vi "stop.vi"(11 "Experience ID":string="Test") -> (0 "error out":errorcluster={"status"=TRUE, "code"=2, "source"="incorrect path for Experience ID"})   [LabVIEW 2020]
uses:
  Configuration/Global_Configurations.vi
panel:
  # "Stop"
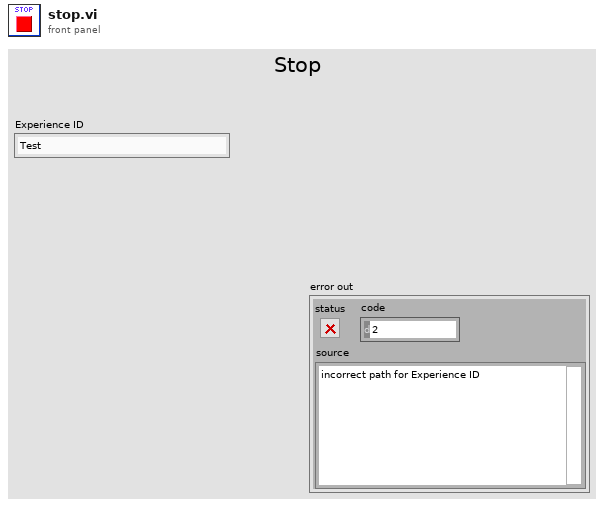
[diagram p1: front panel]
types:
  T1 = enum32{"Bad", "Idle", "Run top level", "Running"}
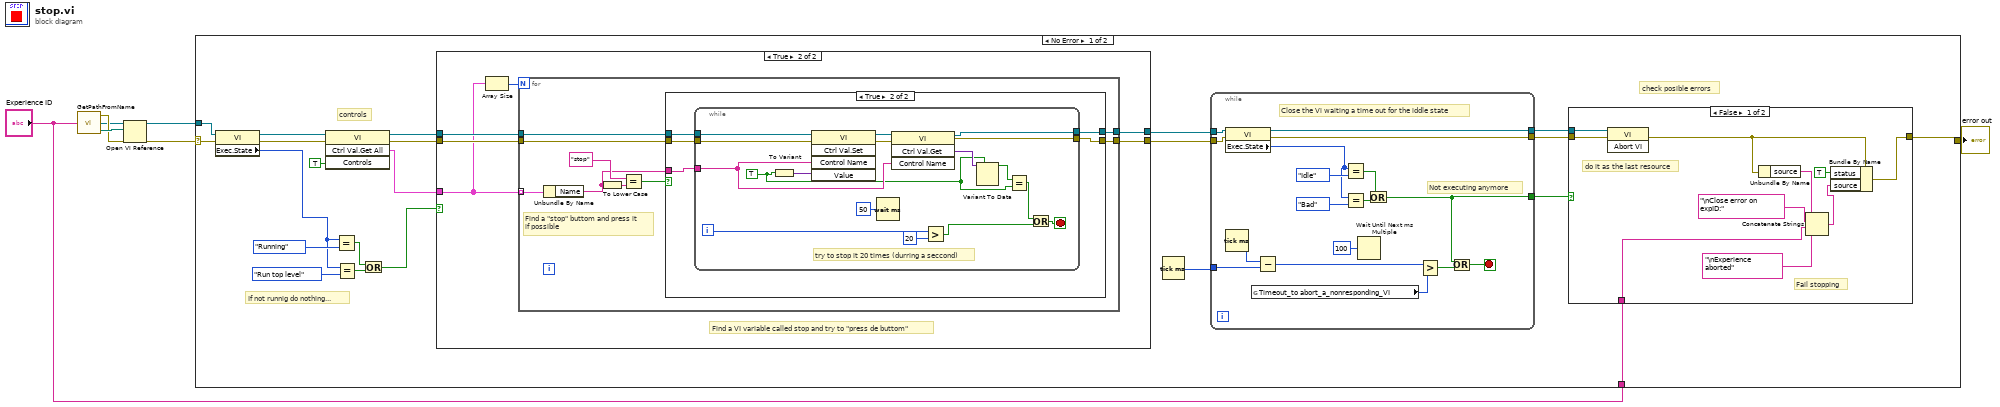
[diagram p0: block diagram]
diagram:
  n1 = call "GetPathFromName.vi"("Experience ID"="Experience ID") -> ("VI_Path"=w7:path, "application reference"=w1:refnum<vi>, "Error out"=w6:errorcluster)  [unwired: 2 in]
  n2 = Open VI Reference(application reference (local)=w1, vi path=w7, error in (no error)=w6) -> (vi reference=w3:refnum<vi>, error out=w4:errorcluster)  [unwired: 3 out]
  n3 = case shown="No Error" w4 {
    selector: w4 -> [w18 w99]
    tunnel: [w15 w99] -> w5
    tunnel: w3 -> [w17 _]
    tunnel: "Experience ID" -> [w14 _]
    frame No Error {
      # "check posible errors"
      # "If not runnig do nothing..."
      # "controls"
      n4 = property class="VI"(reference=w17, error in=w18) -> (reference out=w23:refnum<vi>, error out=w22:errorcluster, "Exec.State"=w16:T1)
      n5 = invoke class="VI" method="Ctrl Val.Get All"(reference=w23, error in=w22, "Controls"=TRUE) -> (reference out=w24:refnum<vi>, error out=w21:errorcluster, "Get All Control Values Variant"=w20:cluster{"Name":string, "Variant Data":variant}[])  [unwired: 1 in, 1 out]
      n6 = Equal?(x=w16, y=T1."Running") -> (x = y?=w28:bool)
      n7 = Equal?(x=w16, y=T1."Run top level") -> (x = y?=w26:bool)
      n8 = Or(x=w28, y=w26) -> (x .or. y?=w19:bool)
      n9 = case shown="True" w19 {
        tunnel: w20 -> [_ w61]
        tunnel: w24 -> [w58 w65]
        tunnel: w21 -> [w59 w64]
        tunnel: [w59 w63] -> w13
        tunnel: [w58 w60] -> w12
        frame False {
        }
        frame True {
          # "Find a VI variable called stop and try to \"press de buttom\""
          n10 = Array Size(array=w61) -> (size(s)=w62:i32)
          n11 = for {
            N: w62 -> [_]
            tunnel: w61 -> [w74] mode=indexing
            tunnel: w65 -> [w72]
            tunnel: w64 -> [w71]
            tunnel: [w69] -> w63
            tunnel: [w66] -> w60
            # "Find a \"stop\" buttom and press it\nif possible"
            n12 = Unbundle By Name(w74) -> ("Name"=w67:string)
            n13 = To Lower Case(string=w67) -> (all lower case string=w68:string)
            n14 = Equal?(x="stop" ("y"), y=w68) -> (x = y?=w73:bool)
            n15 = case shown="True" w73 {
              tunnel: w72 -> [w75 w81]
              tunnel: w71 -> [w76 w80]
              tunnel: [w76 w79] -> w69
              tunnel: w67 -> [_ w78]
              tunnel: [w75 w77] -> w66
              frame False {
              }
              frame True {
                n16 = while {
                  tunnel: w81 -> [w96]
                  tunnel: w80 -> [w98]
                  tunnel: [w83] -> w79
                  tunnel: w78 -> [w88]
                  tunnel: [w82] -> w77
                  i -> [w94]
                  stop <- w95 stop-if-true
                  w85 = TRUE
                  # "try to stop it 20 times (durring a seccond)"
                  n17 = To Variant(anything=w85) -> (Variant=w97:variant)
                  n18 = invoke class="VI" method="Ctrl Val.Set"(reference=w96, error in=w98, "Control Name"=w88, "Value"=w97) -> (reference out=w90:refnum<vi>, error out=w89:errorcluster)  [unwired: 1 in, 3 out]
                  n19 = Wait (ms)(milliseconds to wait=u32 50) -> ()  [unwired: 1 out]
                  n20 = invoke class="VI" method="Ctrl Val.Get"(reference=w90, error in=w89, "Control Name"=w88) -> (reference out=w82:refnum<vi>, error out=w83:errorcluster, "Get Control Value Variant"=w87:variant)  [unwired: 1 in, 1 out]
                  n21 = Greater?(x=w94, y=20) -> (0:w92:bool)
                  n22 = Variant To Data(type=w85, Variant=w87) -> (data=w84:bool)  [unwired: 1 in, 1 out]
                  n23 = Equal?(x=w84, y=w85) -> (x = y?=w86:bool)
                  n24 = Or(x=w86, y=w92) -> (x .or. y?=w95:bool)
                }
              }
            }
          }
        }
      }
      n25 = Tick Count (ms)() -> (millisecond timer value=w11:u32)
      n26 = while {
        tunnel: w12 -> [w46]
        tunnel: [w36] -> w8
        tunnel: [w37] -> w10
        tunnel: [w31] -> w9
        tunnel: w11 -> [w39]
        tunnel: w13 -> [w30]
        stop <- w43 stop-if-true
        # "Not executing anymore"
        # "Close the Vi waiting a time out for the iddle state"
        n27 = property class="VI"(reference=w46, error in=w30) -> (reference out=w36:refnum<vi>, error out=w37:errorcluster, "Exec.State"=w33:T1)
        n28 = Tick Count (ms)() -> (millisecond timer value=w38:u32)
        n29 = global read "Global_Configurations.vi" "Timeout_to abort_a_nonresponding_VI"() -> (w40:u32)
        n30 = Subtract(x=w38, y=w39) -> (x-y=w41:u32)
        n31 = Equal?(x=w33, y=T1."Idle") -> (x = y?=w35:bool)
        n32 = Equal?(x=w33, y=T1."Bad") -> (x = y?=w32:bool)
        n33 = Wait Until Next ms Multiple(millisecond multiple=u32 100) -> ()  [unwired: 1 out]
        n34 = Or(x=w35, y=w32) -> (x .or. y?=w31:bool)
        n35 = Greater?(x=w41, y=w40) -> (0:w42:bool)
        n36 = Or(x=w31, y=w42) -> (x .or. y?=w43:bool)
      }
      n37 = case shown="False" w9 {
        tunnel: [w56 w57] -> w15
        tunnel: w10 -> [w48 w57]
        tunnel: w14 -> [w51 _]
        tunnel: w8 -> [w49 _]
        frame False {
          # "do it as the last resource"
          # "Fail stopping"
          n38 = invoke class="VI" method="Abort VI"(reference=w49, error in=w48) -> (error out=w50:errorcluster)  [unwired: 1 in, 2 out]
          n39 = Unbundle By Name(w50) -> ("source"=w53:string)
          n40 = Concatenate Strings(w53, "\nClose error on expID:" ("string"), w51, "\nExperience aborted" ("string")) -> (w54:string)
          n41 = Bundle By Name(cluster=w50, "status"=TRUE, "source"=w54) -> (w56:errorcluster)
        }
        frame True {
          # "ok"
        }
      }
    }
    frame Error {
    }
  }
  "error out" <- w5
